vi "电机使能.vi"() -> (0 "运控模式报文发送":string)   [LabVIEW 2023]
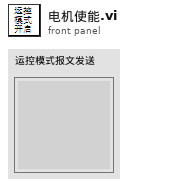
[diagram p1: front panel]
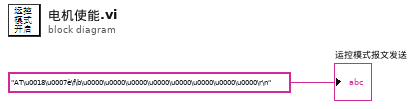
[diagram p0: block diagram]
diagram:
  "运控模式报文发送" <- "AT\u0018\u0007è\f\b\u0000\u0000\u0000\u0000\u0000\u0000\u0000\u0000\r\n"
